vi "Main.vi"() -> ()   [LabVIEW 2019]
uses:
  <vilib>/myRIO/Instrument Drivers/Onboard IO/I2C/typedefs/I2C User Configuration.ctl
  <vilib>/myRIO/Instrument Drivers/Onboard IO/I2C/typedefs/I2C Transfer Rate.ctl
  <vilib>/Platform/TimedLoop/XDataNode/timing_clust.ctl
  <vilib>/Platform/TimedLoop/XDataNode/nitl_modes.ctl
  <vilib>/Platform/TimedLoop/XDataNode/wakeup.ctl
  <vilib>/myRIO/Common/Instrument Driver Framework/myRIO v1.0/DIO/vis/myRIO v1.1 Open DIO.vi
  <vilib>/myRIO/Common/Instrument Driver Framework/myRIO v1.0/I2C/vis/myRIO v1.1 Open I2C.vi
  <vilib>/myRIO/Common/Instrument Driver Framework/myRIO v1.0/UART/vis/myRIO v1.0 Close UART.vi
  <vilib>/myRIO/Common/Instrument Driver Framework/Utilities/vis/Validate Channels.vi
  <vilib>/myRIO/Common/Instrument Driver Framework/myRIO v1.0/DIO/vis/myRIO v1.0 Reserve DIO.vi
  <vilib>/myRIO/Common/Instrument Driver Framework/myRIO v1.0/I2C/vis/myRIO v1.0 Reserve I2C.vi
  <vilib>/myRIO/Common/Instrument Driver Framework/myRIO v1.0/Resource Manager/vis/myRIO v1.0 Reserve Channel List.vi
  <vilib>/myRIO/Common/Instrument Driver Framework/myRIO v1.0/DIO/vis/myRIO v1.0 Build MUX Configuration DIO.vi
  <vilib>/myRIO/Common/Instrument Driver Framework/myRIO v1.0/I2C/vis/myRIO v1.0 Build MUX Configuration I2C.vi
  <vilib>/myRIO/Common/Instrument Driver Framework/myRIO v1.0/Resource Manager/vis/myRIO v1.0 Reserve Channel.vi
  <vilib>/myRIO/Common/Instrument Driver Framework/myRIO v1.0/Resource Manager/vis/myRIO v1.0 Unreserve Channel.vi
  <vilib>/myRIO/Common/Instrument Driver Framework/myRIO v1.0/Resource Manager/vis/myRIO v1.0 Create Configuration List.vi
  <vilib>/myRIO/Common/Instrument Driver Framework/myRIO v1.0/Resource Manager/vis/myRIO v1.0 Build Mutex Name.vi
  <vilib>/Utility/VariantDataType/GetNumericInfo.vi
  <vilib>/Utility/error.llb/Error Cluster From Error Code.vi
  <vilib>/myRIO/Common/Instrument Driver Framework/myRIO v1.0/myRIO v1.1 Open.vi
  <vilib>/myRIO/Common/Instrument Driver Framework/Utilities/vis/IO Manager.vi
  <vilib>/myRIO/Common/Instrument Driver Framework/Utilities/vis/Configuration Manager.vi
  <vilib>/myRIO/Common/Instrument Driver Framework/myRIO v1.0/Resource Manager/vis/myRIO v1.0 Configure IO.vi
  <vilib>/myRIO/Common/Instrument Driver Framework/myRIO v1.0/myRIO v1.0 Close.vi
  <vilib>/myRIO/Common/Instrument Driver Framework/myRIO v1.0/I2C/vis/myRIO v1.0 Configure I2C.vi
  <vilib>/myRIO/Common/Instrument Driver Framework/myRIO v1.0/I2C/vis/myRIO v1.0 Write I2C.vi
  <vilib>/myRIO/Common/Instrument Driver Framework/myRIO v1.0/DIO/vis/myRIO v1.0 Read DIO.vi
  <vilib>/myRIO/Common/Instrument Driver Framework/myRIO v1.0/I2C/vis/myRIO v1.0 Read I2C.vi
  <vilib>/myRIO/Common/Instrument Driver Framework/Utilities/vis/FPGA Ref Manager.vi
  <vilib>/myRIO/Common/Instrument Driver Framework/myRIO v1.0/myRIO v1.0 Reset FPGA.vi
  <vilib>/myRIO/Common/Instrument Driver Framework/myRIO v1.0/IRQ/vis/myRIO v1.0 IRQ Info FGV.vi
  <vilib>/myRIO/Common/Instrument Driver Framework/myRIO v1.0/IRQ/vis/myRIO v1.0 Timer IRQ Info FGV.vi
  <vilib>/myRIO/Common/Instrument Driver Framework/myRIO v1.0/IRQ/vis/myRIO v1.0 ISR Agent.vi
  <vilib>/myRIO/Instrument Drivers/Utilities/vis/Reset Index.vi
  <vilib>/myRIO/Common/Instrument Driver Framework/myRIO v1.0/Resource Manager/vis/myRIO v1.0 Block Write Resource Manager.vi
  <vilib>/platform/TimedLoop/XDataNode/XDataNode.xnode
  <vilib>/myRIO/Instrument Drivers/Utilities/Utilities.lvlib
  <vilib>/myRIO/Instrument Drivers/Onboard IO/I2C/I2C.lvlib
  <vilib>/myRIO/Instrument Drivers/Onboard IO/DIO/DIO.lvlib
  <vilib>/Platform/TimedLoop/XDataNode/XDNodeRunTimeDep.lvlib
panel:
  in  "Y degrees  offset trim angle":sgl=0.95000005 min=-2 max=2 step=0.01
  out "XY Graph":cluster{"t":dbl[], "t":dbl[]}(graph)={"t"=[-97.99660335803118, -96.99663801764311, -95.99667267725503, -94.99670733686696, -93.99674199647889, -92.99677665609082, -91.99681131570274, -90.99684597531467, -89.9968806349266, -88.99691529453852, -87.99694995415045, -86.99698461376238, -85.9970192733743, -84.99705393298623, -83.99708859259816, -82.99712325221009, -81.99715791182201, -80.99719257143394, -79.99722723104585, -78.99726189065778, -77.99729655026971, -76.99733120988164, -75.99736586949356, -74.99740052910549, -73.99743518871742, -72.99746984832935, -71.99750450794127, -70.9975391675532, -69.99757382716513, -68.99760848677705, -67.99764314638898, -66.99767780600091, -65.99771246561284, -64.99774712522476, -63.99778178483669, -62.99781644444862, -61.997851104060544, -60.99788576367247, -59.9979204232844, -58.997955082896326, -57.99798974250825, -56.99802440212018, -55.99805906173211, -54.99809372134403, -53.998128380955954, -52.99816304056788, -51.99819770017981, -50.998232359791736, -49.99826701940366, -48.99830167901559, -47.99833633862752, -46.998370998239444, -45.99840565785137, -44.9984403174633, -43.998474977075226, -42.99850963668715, -41.99854429629908, -40.99857895591101, -39.99861361552293, -38.998648275134855, -37.99868293474678, -36.99871759435871, -35.998752253970636, -34.99878691358256, -33.99882157319449, -32.99885623280642, -31.998890892418345, -30.998925552030272, -29.9989602116422, -28.998994871254126, -27.999029530866054, -26.999064190477977, -25.999098850089904, -24.99913350970183, -23.99916816931376, -22.999202828925686, -21.999237488537613, -20.99927214814954, -19.999306807761464, -18.99934146737339, -17.999376126985318, -16.999410786597245, -15.999445446209172, -14.9994801058211, -13.999514765433027, -12.999549425044952, -11.99958408465688, -10.999618744268806, -9.999653403880732, -8.999688063492659, -7.999722723104586, -6.999757382716513, -5.99979204232844, -4.999826701940366, -3.999861361552293, -2.99989602116422, -1.9999306807761466, -0.9999653403880733, 0.0, 0.9999653403880733, 1.9999306807761466, 2.99989602116422, 3.999861361552293, 4.999826701940366, 5.99979204232844, 6.999757382716513, 7.999722723104586, 8.999688063492659, 9.999653403880732, 10.999618744268806, 11.99958408465688, 12.999549425044952, 13.999514765433027, 14.9994801058211, 15.999445446209172, 16.999410786597245, 17.999376126985318, 18.99934146737339, 19.999306807761464, 20.99927214814954, 21.999237488537613, 22.999202828925686, 23.99916816931376, 24.99913350970183, 25.999098850089904, 26.999064190477977, 27.999029530866054, 28.998994871254126, 29.9989602116422, 30.998925552030272, 31.998890892418345, 32.99885623280642, 33.99882157319449, 34.99878691358256, 35.998752253970636, 36.99871759435871, 37.99868293474678, 38.998648275134855, 39.99861361552293, 40.99857895591101, 41.99854429629908, 42.99850963668715, 43.998474977075226, 44.9984403174633, 45.99840565785137, 46.998370998239444, 47.99833633862752, 48.99830167901559, 49.99826701940366, 50.998232359791736, 51.99819770017981, 52.99816304056788, 53.998128380955954, 54.99809372134403, 55.99805906173211, 56.99802440212018, 57.99798974250825, 58.997955082896326, 59.9979204232844, 60.99788576367247, 61.997851104060544, 62.99781644444862, 63.99778178483669, 64.99774712522476, 65.99771246561284, 66.99767780600091, 67.99764314638898, 68.99760848677705, 69.99757382716513, 70.9975391675532, 71.99750450794127, 72.99746984832935, 73.99743518871742, 74.99740052910549, 75.99736586949356, 76.99733120988164, 77.99729655026971, 78.99726189065778, 79.99722723104585, 80.99719257143394, 81.99715791182201, 82.99712325221009, 83.99708859259816, 84.99705393298623, 85.9970192733743, 86.99698461376238, 87.99694995415045, 88.99691529453852, 89.9968806349266, 90.99684597531467, 91.99681131570274, 92.99677665609082, 93.99674199647889, 94.99670733686696, 95.99667267725503, 96.99663801764311, 97.99660335803118, 98.99656869841925, 99.99653403880733], "t"=[0.8159229673880889, 0.8075972228229044, 0.7992714782577197, 0.7909457336925352, 0.7826199891273506, 0.774294244562166, 0.7659684999969815, 0.7576427554317968, 0.7493170108666123, 0.7409912663014278, 0.7326655217362431, 0.7243397771710586, 0.7160140326058739, 0.7076882880406894, 0.6993625434755047, 0.6910367989103202, 0.6827110543451357, 0.674385309779951, 0.6660595652147665, 0.6577338206495819, 0.6494080760843973, 0.6410823315192127, 0.6327565869540281, 0.6244308423888436, 0.616105097823659, 0.6077793532584744, 0.5994536086932898, 0.5911278641281053, 0.5828021195629207, 0.5744763749977361, 0.5661506304325515, 0.5578248858673669, 0.5494991413021824, 0.5411733967369977, 0.5328476521718132, 0.5245219076066286, 0.516196163041444, 0.5078704184762595, 0.4995446739110749, 0.4912189293458903, 0.4828931847807057, 0.4745674402155211, 0.4662416956503365, 0.45791595108515193, 0.4495902065199674, 0.4412644619547828, 0.4329387173895982, 0.4246129728244136, 0.41628722825922904, 0.40796148369404445, 0.39963573912885986, 0.3913099945636753, 0.38298424999849073, 0.37465850543330614, 0.36633276086812155, 0.35800701630293696, 0.3496812717377524, 0.34135552717256784, 0.33302978260738325, 0.32470403804219866, 0.31637829347701407, 0.3080525489118295, 0.2997268043466449, 0.29140105978146036, 0.28307531521627577, 0.2747495706510912, 0.2664238260859066, 0.258098081520722, 0.24977233695553744, 0.24144659239035285, 0.23312084782516826, 0.2247951032599837, 0.2164693586947991, 0.20814361412961452, 0.19981786956442993, 0.19149212499924537, 0.18316638043406078, 0.1748406358688762, 0.16651489130369163, 0.15818914673850704, 0.14986340217332245, 0.14153765760813788, 0.1332119130429533, 0.12488616847776872, 0.11656042391258413, 0.10823467934739955, 0.09990893478221496, 0.09158319021703039, 0.08325744565184581, 0.07493170108666122, 0.06660595652147665, 0.058280211956292065, 0.04995446739110748, 0.041628722825922906, 0.033302978260738324, 0.02497723369555374, 0.016651489130369162, 0.008325744565184581, -0.0, -0.008325744565184581, -0.016651489130369162, -0.02497723369555374, -0.033302978260738324, -0.041628722825922906, -0.04995446739110748, -0.058280211956292065, -0.06660595652147665, -0.07493170108666122, -0.08325744565184581, -0.09158319021703039, -0.09990893478221496, -0.10823467934739955, -0.11656042391258413, -0.12488616847776872, -0.1332119130429533, -0.14153765760813788, -0.14986340217332245, -0.15818914673850704, -0.16651489130369163, -0.1748406358688762, -0.18316638043406078, -0.19149212499924537, -0.19981786956442993, -0.20814361412961452, -0.2164693586947991, -0.2247951032599837, -0.23312084782516826, -0.24144659239035285, -0.24977233695553744, -0.258098081520722, -0.2664238260859066, -0.2747495706510912, -0.28307531521627577, -0.29140105978146036, -0.2997268043466449, -0.3080525489118295, -0.31637829347701407, -0.32470403804219866, -0.33302978260738325, -0.34135552717256784, -0.3496812717377524, -0.35800701630293696, -0.36633276086812155, -0.37465850543330614, -0.38298424999849073, -0.3913099945636753, -0.39963573912885986, -0.40796148369404445, -0.41628722825922904, -0.4246129728244136, -0.4329387173895982, -0.4412644619547828, -0.4495902065199674, -0.45791595108515193, -0.4662416956503365, -0.4745674402155211, -0.4828931847807057, -0.4912189293458903, -0.4995446739110749, -0.5078704184762595, -0.516196163041444, -0.5245219076066286, -0.5328476521718132, -0.5411733967369977, -0.5494991413021824, -0.5578248858673669, -0.5661506304325515, -0.5744763749977361, -0.5828021195629207, -0.5911278641281053, -0.5994536086932898, -0.6077793532584744, -0.616105097823659, -0.6244308423888436, -0.6327565869540281, -0.6410823315192127, -0.6494080760843973, -0.6577338206495819, -0.6660595652147665, -0.674385309779951, -0.6827110543451357, -0.6910367989103202, -0.6993625434755047, -0.7076882880406894, -0.7160140326058739, -0.7243397771710586, -0.7326655217362431, -0.7409912663014278, -0.7493170108666123, -0.7576427554317968, -0.7659684999969815, -0.774294244562166, -0.7826199891273506, -0.7909457336925352, -0.7992714782577197, -0.8075972228229044, -0.8159229673880889, -0.8242487119532735, -0.8325744565184581]}
  out "Y displacement degrees from complementary filter":dbl=-0.47703553619064704 format="%#_5g"
  in  "Y offset trim gyro velocity":i16=50
  out "Z acc":i16=14868
  out "X acc":i16=-1088
  out "Y Gyro rate":i16=16
  in  "?":bool
  # "MPU6050 with\nComplementary Filter"
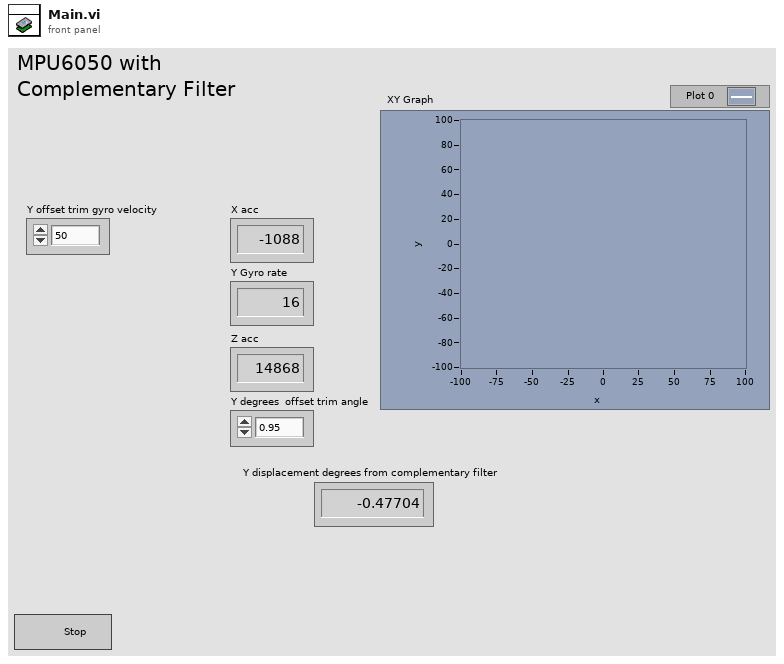
[diagram p1: front panel]
types:
  T1 = typedef "I2C.lvlib/I2C User Configuration.ctl" = cluster{"I2C Transfer Rate":T2}
  T2 = typedef "I2C.lvlib/I2C Transfer Rate.ctl" = enum16{"Standard mode (100 kbps)", "Fast mode (400 kbps)"}
  T3 = typedef "I2C.lvlib/I2C Reference.ctl" = cluster{"myRIO Reference":T4, "I2C Channels Enum":T8, "I2C Configuration":T9}
  T4 = typedef "myRIO Generic Hardware Reference.ctl" = cluster{"myRIO Model":T5, "myRIO Hardware Reference":T6}
  T5 = typedef "Hardware Version Enum.ctl" = enum16{"Unknown", "myRIO-1900", "myRIO-1950", "roboRIO", "NI ELVIS RIO CM", "ELVIS III"}
  T6 = typedef "myRIO v1.0 Reference.ctl" = cluster{"Generic FPGA Reference":T7, "Allow multiple opens":bool}
  T7 = typedef "Generic FPGA Reference.ctl" = refnum<k20>
  T8 = typedef "I2C Channels Enum.ctl" = enum16{"Not Connected", "A/I2C", "B/I2C", "I2C/I2C"}
  T9 = typedef "I2C.lvlib/I2C Configuration.ctl" = cluster{"I2C Transfer Rate":T2}
  T10 = typedef "DIO.lvlib/DIO Reference.ctl" = cluster{"myRIO Reference":T4, "DIO Channels List":T11}
  T11 = typedef "DIO Channels List.ctl" = T12[]
  T12 = typedef "DIO Channels Enum.ctl" = enum16{"Not Connected", "C/DIO0", "C/DIO1", "C/DIO2", "C/DIO3", "C/DIO4", "C/DIO5", "C/DIO6", "C/DIO7", "A/DIO0", "A/DIO1", "A/DIO2", "A/DIO3", "A/DIO4", "A/DIO5", "A/DIO6", "A/DIO7", "A/DIO8", "A/DIO9", "A/DIO10", "A/DIO11", "A/DIO12", "A/DIO13", "A/DIO14", "A/DIO15", "A/DIO16", "A/DIO17", "A/DIO18", "A/DIO19", "B/DIO0", "B/DIO1", "B/DIO2", "B/DIO3", "B/DIO4", "B/DIO5", "B/DIO6", "B/DIO7", "B/DIO8", "B/DIO9", "B/DIO10", "B/DIO11", "B/DIO12", "B/DIO13", "B/DIO14", "B/DIO15", "B/DIO16", "B/DIO17", "B/DIO18", "B/DIO19", "LED0", "LED1", "LED2", "LED3", "Button0", "DIO/DIO0", "DIO/DIO1", "DIO/DIO2", "DIO/DIO3", "DIO/DIO4", "DIO/DIO5", "DIO/DIO6", "DIO/DIO7", "DIO/DIO8", "DIO/DIO9", "SPI/CS0", "SPI/CS1", "SPI/CS2", "SPI/CS3", "LED RADIO (Green)", "LED RADIO (Red)", "LED COMM (Green)", "LED COMM (Red)", "LED MODE (Green)", "LED MODE (Red)"}
  T13 = typedef "XDNodeRunTimeDep.lvlib/timing_clust.ctl" = cluster{"Expected End [f-1]":u64, "Actual End [f-1]":u64, "Finished Late? [f-1]":bool, "Expected End [i-1]":u64, "Actual End [i-1]":u64, "Finished Late? [i-1]":bool, "Expected Start [i]":u64, "Actual Start [i]":u64, "Expected Start [f]":u64, "Actual Start [f]":u64, "Source Name":string, "Structure Name":string, "Period":i64, "Deadline":i64, "Offset":i64, "Start":i64, "Priority":i32, "Timeout":i32, "Mode":T14, "Wakeup Reason":T15, "Error":errorcluster, "Source Type":string, "Secondary Source Type":string, "Global End Time":u64, "Global Start Time":u64, "Frame Duration":u64, "Iteration Duration":u64, "Assigned CPU":i32, "I/O Scan Engine Mode":u32}
  T14 = typedef "XDNodeRunTimeDep.lvlib/nitl_modes.ctl" = enum32{"No Change", "Process missed periods, maintain original phase", "Discard missed periods, maintain original phase", "Process missed periods, ignore original phase", "Discard missed periods, ignore original phase"}
  T15 = typedef "XDNodeRunTimeDep.lvlib/wakeup.ctl" = enum32{"Normal", "Aborted", "Asynchronous wakeup", "Timing source error", "Timed loop error", "Timeout"}
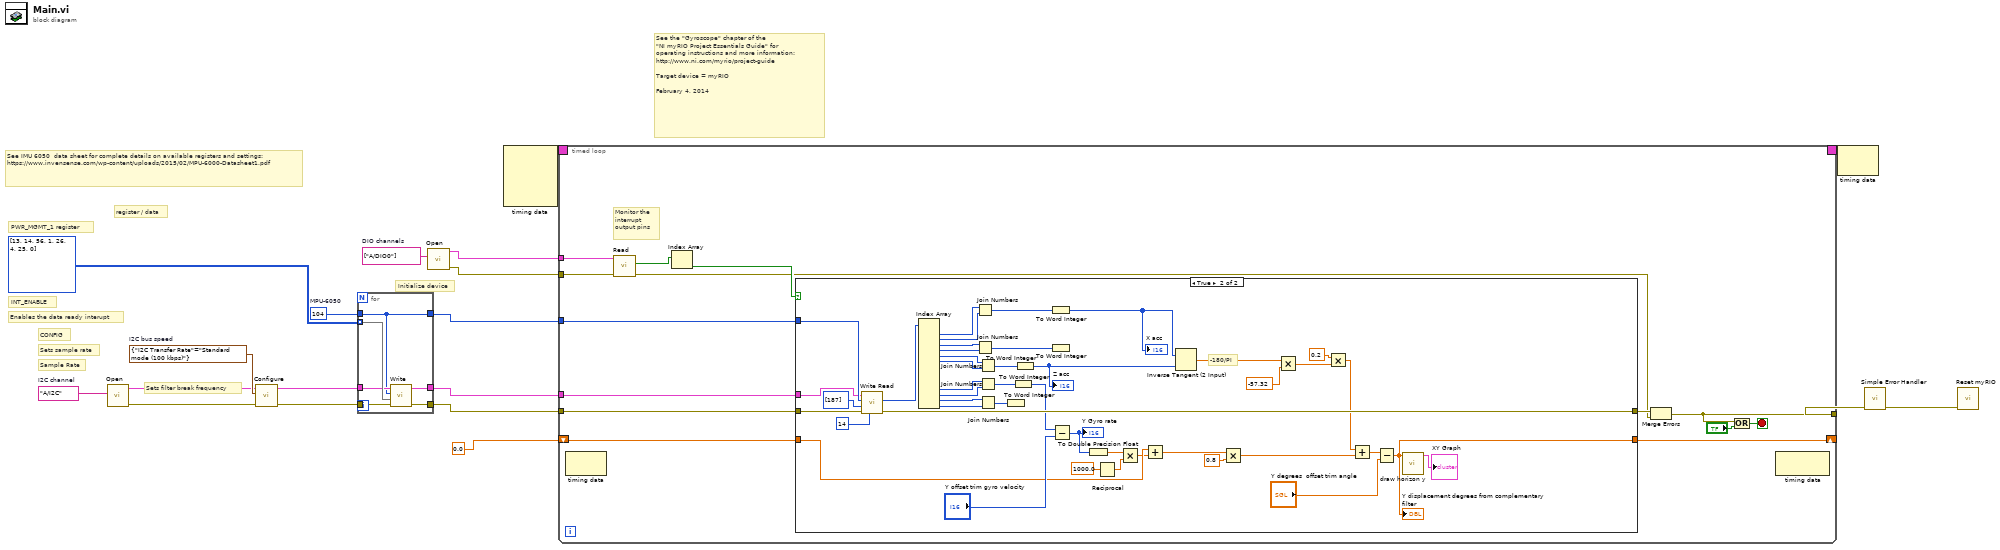
[diagram p0: block diagram]
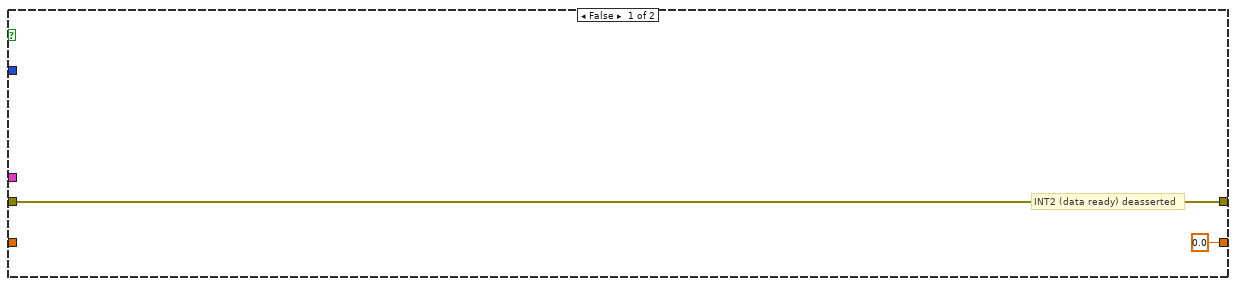
[diagram p2: hidden frame]
diagram:
  w6 = tag[] ["A/DIO0"]  # DIO channels
  w17 = T1 {"I2C Transfer Rate"=enum."Standard mode (100 kbps)"}  # I2C bus speed
  w2 = tag "A/I2C"  # I2C channel
  w8 = u8 104  # MPU-6050
  # "Sets sample rate"
  # "Sample Rate"
  # "Sets filter break frequency"
  # "CONFIG"
  # "INT_ENABLE"
  # "Enables the data ready interupt"
  # "See the \"Gyroscope\" chapter of the\n\"NI myRIO Project Essentials Guide\" for\noperating instructions and more information: \nhttp://www.ni.com/myrio/project-guide\n\nTarget device = myRIO\n\nFebruary 4, 2014"
  # "PWR_MGMT_1 register"
  # "Initialize device"
  # "See IMU 6050  data sheet for complete details on available registers and settings:\nhttps://www.invensense.com/wp-content/uploads/2015/02/MPU-6000-Datasheet1.pdf"
  # "register / data"
  n1 = call <vilib>:"Open.vi"("Channel Name"=w2) -> ("error out"=w15:errorcluster, "I2C Ref Out"=w16:T3)  [unwired: 9 in]
  n2 = call <vilib>:"Configure.vi"("error in (no error)"=w15, "I2C User Configuration"=w17, "I2C Ref In"=w16) -> ("error out"=w9:errorcluster, "I2C Ref Out"=w10:T3)  [unwired: 7 in]
  n3 = for {
    tunnel: [w25] -> w14
    tunnel: [w24] -> w13
    tunnel: [w20] -> w12
    tunnel: u8[][] [[13, 14], [56, 1], [26, 4], [25, 0]] ("Bytes to Write") -> [w23] mode=indexing
    tunnel: w10 -> [w22]
    tunnel: w9 -> [w21]
    tunnel: w8 -> [w20]
    n4 = call <vilib>:"Write.vi"("error in (no error)"=w21, "Bytes to Write"=w23, "Slave Address (7-bit)"=w20, "I2C Ref In"=w22) -> ("error out"=w25:errorcluster, "I2C Ref Out"=w24:T3)  [unwired: 6 in]
  }
  n5 = call <vilib>:"Open.vi"("Channel Names"=w6) -> ("error out"=w7:errorcluster, "DIO Ref Out"=w3:T10)  [unwired: 9 in]
  n6 = node-c288() -> (w5:T13)  [unwired: 4 in]
  n7 = timed-loop {
    tunnel: [w30] -> w18
    tunnel: w12 -> [w35]
    tunnel: w14 -> [w37]
    tunnel: w13 -> [w36]
    tunnel: w7 -> [w34]
    timing: w5 -> [_]
    timing-out: [_] -> w4
    tunnel: w3 -> [w29]
    shift-right: [w27] -> _
    shift-left: 0.0 -> [w26]
    stop <- w39 stop-if-true
    # "Monitor the\ninterrupt\noutput pins"
    n8 = node-c288() -> ()  [unwired: 1 in, 1 out]
    n9 = call <vilib>:"Read.vi"("error in (no error)"=w34, "DIO Ref In"=w29) -> ("error out"=w28:errorcluster, "Values"=w31:bool[])  [unwired: 7 in, 1 out]
    n10 = Index Array "Index Array"(array=w31) -> (element=w32:bool)  [unwired: 1 in]
    n11 = case shown="True" w32 {
      tunnel: w37 -> [w43 w79]
      tunnel: w36 -> [_ w80]
      tunnel: w35 -> [_ w83]
      tunnel: [w43 w82] -> w33
      tunnel: [0.0 w45] -> w27
      tunnel: w26 -> [_ w56]
      frame False {
        # "INT2 (data ready) deasserted"
      }
      frame True {
        # "-180/PI"
        n12 = call <vilib>:"Write Read.vi"("Byte Count"=u32 14, "error in (no error)"=w79, "Bytes to Write"=u8[] [187], "Slave Address (7-bit)"=w83, "I2C Ref In"=w80) -> ("error out"=w82:errorcluster, "Bytes Read"=w81:u8[])  [unwired: 3 in, 1 out]
        n13 = Index Array "Index Array"(array=w81) -> (element #1=w78:u8, element #2=w77:u8, element #3=w64:u8, element #4=w63:u8, element #5=w76:u8, element #6=w75:u8, element #11=w74:u8, element #12=w73:u8, element #13=w72:u8, element #14=w71:u8)  [unwired: 14 in, 4 out]
        n14 = Join Numbers(hi=w78, lo=w77) -> ((hi.lo)=w87:u16)
        n15 = Join Numbers(hi=w64, lo=w63) -> ((hi.lo)=w62:u16)
        n16 = Join Numbers(hi=w76, lo=w75) -> ((hi.lo)=w86:u16)
        n17 = Join Numbers(hi=w74, lo=w73) -> ((hi.lo)=w70:u16)
        n18 = Join Numbers(hi=w72, lo=w71) -> ((hi.lo)=w69:u16)
        n19 = To Word Integer(number=w69) -> ()  [unwired: 1 out]
        n20 = To Word Integer(number=w70) -> (16bit integer=w66:i16)
        n21 = To Word Integer(number=w86) -> (16bit integer=w61:i16)
        "Z acc" <- w61
        n22 = To Word Integer(number=w87) -> (16bit integer=w60:i16)
        "X acc" <- w60
        n23 = To Word Integer(number=w62) -> ()  [unwired: 1 out]
        n24 = Subtract(x=w66, y="Y offset trim gyro velocity") -> (x-y=w58:i16)
        "Y Gyro rate" <- w58
        n25 = To Double Precision Float(number=w58) -> (double precision float=w55:dbl)
        n26 = Reciprocal(x=1000.0 ("dt")) -> (1/x=w53:dbl)
        n27 = Multiply(x=w55, y=w53) -> (x*y=w54:dbl)
        n28 = Add(x=w56, y=w54) -> (x+y=w57:dbl)
        n29 = Inverse Tangent (2 Input)(1:w61, 2:w60) -> (0:w68:dbl)
        n30 = Multiply(x=w57, y=0.8) -> (x*y=w49:dbl)
        n31 = Multiply(x=w68, y=-57.32) -> (x*y=w52:dbl)
        n32 = Multiply(x=0.2, y=w52) -> (x*y=w50:dbl)
        n33 = Add(x=w50, y=w49) -> (x+y=w47:dbl)
        n34 = Subtract(x=w47, y="Y degrees  offset trim angle") -> (x-y=w45:dbl)
        "Y displacement degrees from complementary filter" <- w45
        n35 = call "draw horizon y.vi"("angle in degrees in"=w45) -> ("x-y graph"=→"XY Graph":cluster{"t":dbl[], "t":dbl[]})  [unwired: 10 in]
      }
    }
    n36 = Merge Errors "Merge Errors"(w33, w28) -> (w30:errorcluster)
    n37 = Or(x=w30, y="?") -> (x .or. y?=w39:bool)
    n38 = node-c288() -> ()  [unwired: 1 in, 1 out]
  }
  n39 = node-c288(w4) -> ()  [unwired: 1 out]
  n40 = call <vilib>:"Simple Error Handler.vi"("error in (no error)"=w18) -> ("error out"=w19:errorcluster)  [unwired: 4 in, 4 out]
  n41 = call <vilib>:"Reset myRIO.vi"("error in (no error)"=w19) -> ()  [unwired: 10 in, 1 out]
